vi "Write Charact Data Array.vi"(8 "error in (no error)":errorcluster, 10 "Charact Data Array":T1[](array[typedef]), 11 "Vector Path in":refnum<class "Vector Abstract Path.lvclass">) -> (0 "error out":errorcluster, 3 "Vector Path out":refnum<class "Vector Abstract Path.lvclass">)   [LabVIEW 2023, in "RFFixtureCharact.Public.lvlib" / "Vector Abstract Path.lvclass"]
uses:
  Vector Abstract Path.lvclass
  Instruments/Cal Standard/Type Definitions/One-Port Charact Data.ctl
  Instruments/Cal Standard/Type Definitions/Standard Type.ctl
  Vector Abstract Path.lvclass/Vector Abstract Path.ctl
  Instruments/RFFixtureCharact.Instruments.lvlib
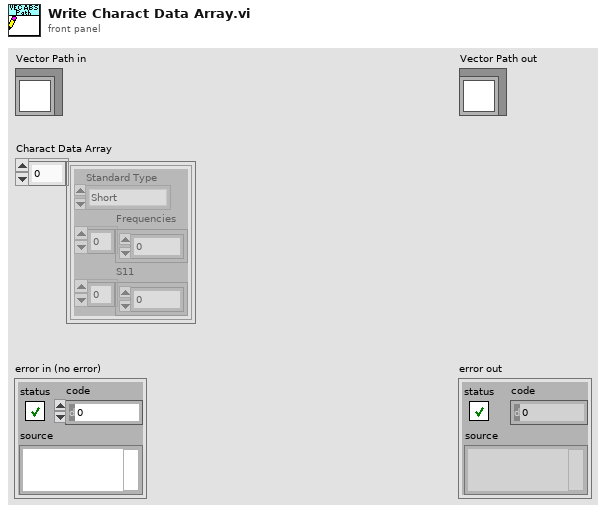
[diagram p1: front panel]
types:
  T1 = typedef "RFFixtureCharact.Instruments.lvlib/One-Port Charact Data.ctl" = cluster{"Standard Type":T2, "Frequencies":dbl[], "S11":cdb[]}
  T2 = typedef "RFFixtureCharact.Instruments.lvlib/Standard Type.ctl" = enum16{"Short", "Open", "Load", "PowerMeter", "None"}
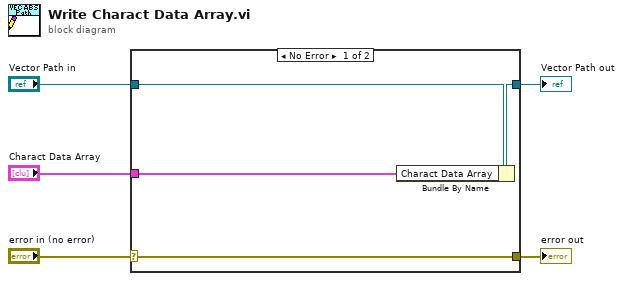
[diagram p0: block diagram]
diagram:
  n1 = case shown="No Error" "error in (no error)" {
    selector: "error in (no error)" -> [w9 w10]
    tunnel: [w9 w10] -> w4
    tunnel: [w7 w11] -> w2
    tunnel: "Vector Path in" -> [w8 w11]
    tunnel: "Charact Data Array" -> [w6 _]
    frame No Error {
      n2 = Bundle By Name(cluster=w8, "Charact Data Array"=w6) -> (w7:refnum<class "Vector Abstract Path.lvclass">)
    }
    frame Error {
    }
  }
  "error out" <- w4
  "Vector Path out" <- w2
